vi "Write position.vi"(8 "error in (no error)":errorcluster, 10 "position":T1, 11 "GObject in":refnum<class "GObject.lvclass">) -> (0 "error out":errorcluster, 3 "GObject out":refnum<class "GObject.lvclass">)   [LabVIEW 2023, in "TLC_Scripto.lvlib" / "GObject.lvclass"]
uses:
  GObject.lvclass
  <vilib>/Utility/miscctls.llb/LVPositionTypeDef.ctl
  Read GObjectRef.vi
  GObject.lvclass/GObject.ctl
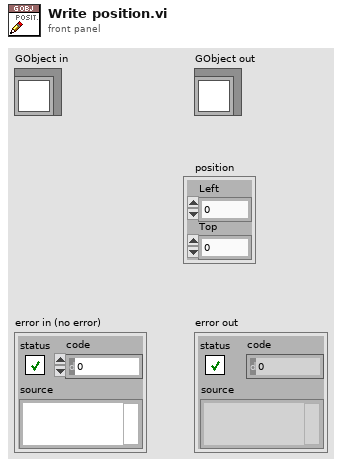
[diagram p1: front panel]
types:
  T1 = typedef "LVPositionTypeDef.ctl" = cluster{"Left":i32, "Top":i32}
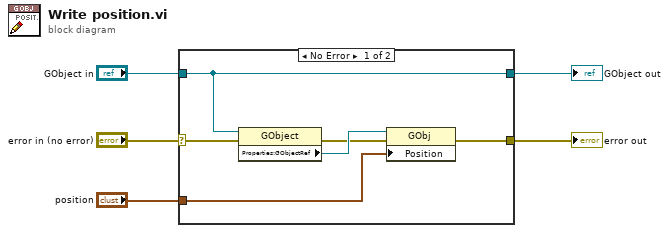
[diagram p0: block diagram]
diagram:
  n1 = case shown="No Error" "error in (no error)" {
    selector: "error in (no error)" -> [w8 w13]
    tunnel: [w7 w13] -> w4
    tunnel: [w11 w12] -> w2
    tunnel: "GObject in" -> [w11 w12]
    tunnel: "position" -> [w6 _]
    frame No Error {
      n2 = property class="GObject"(reference=w11, error in=w8) -> (error out=w9:errorcluster, "Properties:GObjectRef"=w10:refnum<vi>)  [unwired: 1 out]
      n3 = property class="GObj"(reference=w10, error in=w9, "Position"=w6) -> (error out=w7:errorcluster)  [unwired: 1 out]
    }
    frame Error {
    }
  }
  "error out" <- w4
  "GObject out" <- w2
